vi "GetAllLVFilesForLibCheck.vi"(8 "error in (no error)":errorcluster) -> (0 "error out":errorcluster, 3 "LV File paths (VIs, CTLs, LVCLASSes)":path[](array[path]))   [LabVIEW 2019, in "Hawkeye.lvlib"]
uses:
  Hawkeye.lvlib
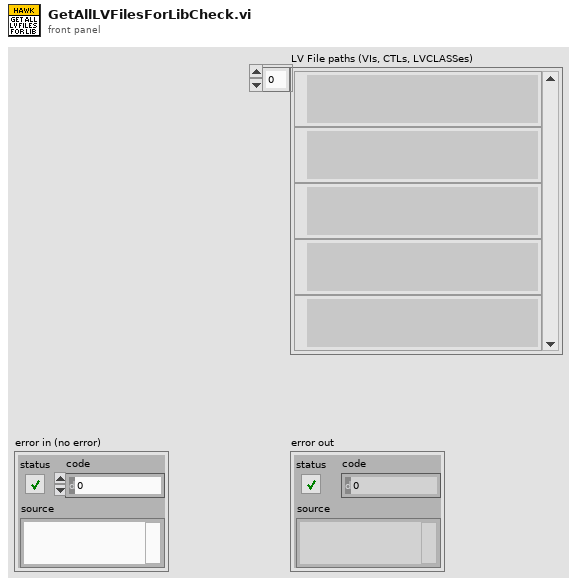
[diagram p1: front panel]
types:
  T1 = typedef "Hawkeye.lvlib/HawkeyePathConfigs.ctl" = cluster{"GlobalIncludePaths":path[], "GlobalExcludePaths":path[], "BuildSpecsIncludePaths":path[], "ActualDepsIncludePaths":path[], "WorkspacePath":path, "SourceFolderPaths":path[], "ChangedFilesLogpaths":map{string, path}}
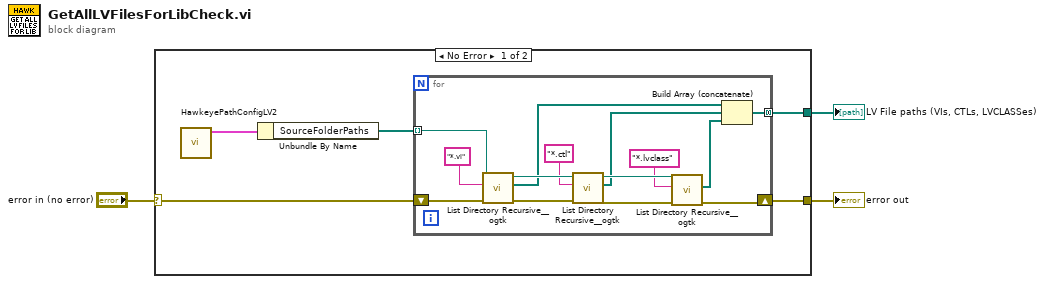
[diagram p0: block diagram]
diagram:
  n1 = case shown="No Error" "error in (no error)" {
    selector: "error in (no error)" -> [w8 w23]
    tunnel: [w6 w23] -> w2
    tunnel: [w4 _] -> w1
    frame No Error {
      n2 = call "HawkeyePathConfigLV2.vi"() -> ("Hawkeye Path Config Out"=w5:T1)  [unwired: 11 in]
      n3 = Unbundle By Name(w5) -> ("SourceFolderPaths"=w7:path[])
      n4 = for {
        shift-right: [w9] -> w6
        shift-left: w8 -> [w22]
        tunnel: w7 -> [w20] mode=indexing
        tunnel: [w10] -> w4 mode=concatenating
        n5 = call <userlib>:"List Directory Recursive__ogtk.vi"("error in (no error)"=w22, "pattern"="*.vi", "Path"=w20) -> ("error out"=w19:errorcluster, "file paths"=w13:path[], "dup Path"=w18:path)  [unwired: 5 in, 1 out]
        n6 = call <userlib>:"List Directory Recursive__ogtk.vi"("error in (no error)"=w19, "pattern"="*.ctl", "Path"=w18) -> ("error out"=w14:errorcluster, "file paths"=w12:path[], "dup Path"=w16:path)  [unwired: 5 in, 1 out]
        n7 = call <userlib>:"List Directory Recursive__ogtk.vi"("error in (no error)"=w14, "pattern"="*.lvclass", "Path"=w16) -> ("error out"=w9:errorcluster, "file paths"=w11:path[])  [unwired: 5 in, 2 out]
        n8 = Build Array (concatenate)(w13, w12, w11) -> (w10:path[])
      }
    }
    frame Error {
      # "Error"
    }
  }
  "error out" <- w2
  "LV File paths (VIs, CTLs, LVCLASSes)" <- w1
